vi "LogFile Kopfzeile eintragen.vi"() -> (2 "LogFile Kopfzeile":string[][](array[string]))   [LabVIEW 2020, in "LogKonfig.lvlib"]
uses:
  LogKonfig.lvlib
  FT-IR/FGV FT-IR Gasliste Aktionen.ctl
  Log Sequence FGV Aktion.ctl
  Sprachverwaltung/FGV Aktion Tabelle zerlegen.ctl
  FT-IR/FT-IR.lvlib
  Sprachverwaltung/Sprachverwaltung.lvlib
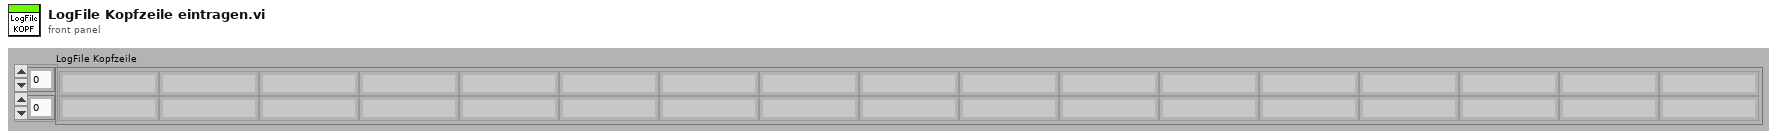
[diagram p1: front panel]
types:
  T1 = typedef "Sprachverwaltung.lvlib/FGV Aktion Tabelle zerlegen.ctl" = enum16{"laden", "vereinzeln", "speichern"}
  T2 = typedef "LogKonfig.lvlib/Log Sequence FGV Aktion.ctl" = enum16{"initialisieren", "lesen", "schreiben", "laden", "speichern", "übertragen"}
  T3 = typedef "FT-IR.lvlib/FGV FT-IR Gasliste Aktionen.ctl" = enum16{"lesen", "Gasliste FT-IR", "Gasliste ausgelesen", "laden", "speichern", "löschen"}
  T4 = cluster{"Index Array":i32[], "Namen Array":string[], "Spektrum File Name":bool}
  T5 = typedef "String - Ausgabefeld.ctl" = string
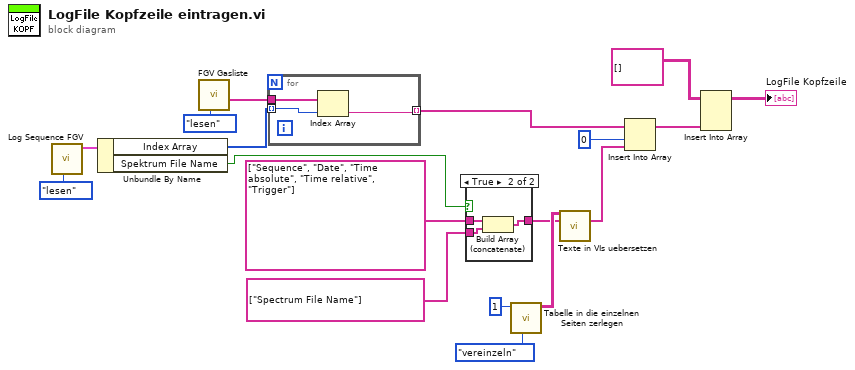
[diagram p0: block diagram]
diagram:
  n1 = call "Log Sequence FGV.vi"("Aktion"=Log_Sequence_FGV_Aktion."lesen") -> ("Cluster (out)"=w13:T4)  [unwired: 10 in]
  n2 = Unbundle By Name(w13) -> ("Index Array"=w12:i32[], "Spektrum File Name"=w2:bool)
  n3 = call "FGV Gasliste.vi"("Aktionen"=FGV_FT-IR_Gasliste_Aktionen."lesen") -> ("Aktuelle Gasliste gesamt"=w11:T5[])  [unwired: 8 in, 2 out]
  n4 = for {
    tunnel: w12 -> [w20] mode=indexing
    tunnel: w11 -> [w21]
    tunnel: [w19] -> w9 mode=indexing
    n5 = Index Array(array=w21, index=w20) -> (element=w19:T5)
  }
  n6 = case shown="True" w2 {
    tunnel: string[] ["Sequence", "Date", "Time absolute", "Time relative", "Trigger"] -> [w22 w25]
    tunnel: [w22 w24] -> w3
    tunnel: string[] ["Spectrum File Name"] -> [_ w23]
    frame False {
    }
    frame True {
      n7 = Build Array (concatenate)(w25, w23) -> (w24:string[])
    }
  }
  n8 = call "Tabelle in die einzelnen Seiten zerlegen.vi"("Aktion"=FGV_Aktion_Tabelle_zerlegen."vereinzeln", "Index (Seite)"=1) -> ("Sprachliste"=w5:string[][])  [unwired: 7 in, 2 out]
  n9 = call "Texte in VIs uebersetzen.vi"("Sprachliste"=w5, "String-Array zum Übersetzen"=w3) -> ("String-Array zum Übersetzen"=w4:string[])  [unwired: 9 in, 4 out]
  n10 = Insert Into Array(array=w9, index=0 ("Index"), new element=w4) -> (w17:T5[])
  n11 = Insert Into Array(array=string[][] [] ("Angehängtes Array"), new element=w17) -> (→"LogFile Kopfzeile":string[][])  [unwired: 2 in]
